vi "Get Resource Path.vi"(8 "Error In":errorcluster, 11 "Resource Filename":string="mine.PNG") -> (0 "Error Out":errorcluster, 3 "Resource Path":path)   [LabVIEW 2011]
doc: "Takes a filename, including file extension, of a file in the Resources directory of the built project and returns a filepath to that resource."
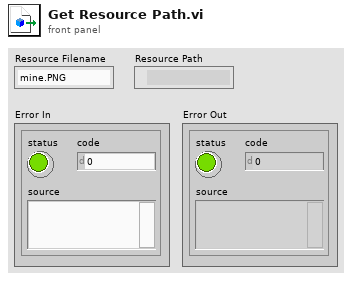
[diagram p1: front panel]
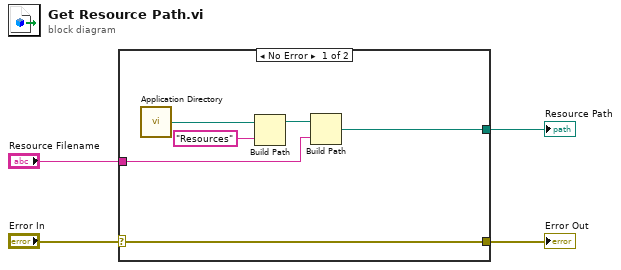
[diagram p0: block diagram]
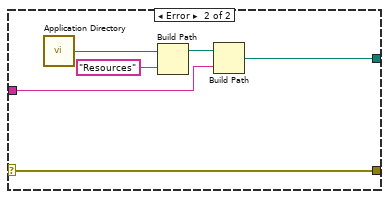
[diagram p2: hidden frame]
diagram:
  n1 = case shown="No Error" "Error In" {
    selector: "Error In" -> [w6 w11]
    tunnel: "Resource Filename" -> [w7 w12]
    tunnel: [w6 w11] -> w2
    tunnel: [w5 w13] -> w1
    frame No Error {
      n2 = call <vilib>:"Application Directory.vi"() -> ("Application Directory"=w9:path)
      n3 = Build Path(base path=w9, name or relative path="Resources") -> (appended path=w8:path)
      n4 = Build Path(base path=w8, name or relative path=w7) -> (appended path=w5:path)
    }
    frame Error {
      n5 = call <vilib>:"Application Directory.vi"() -> ("Application Directory"=w15:path)
      n6 = Build Path(base path=w15, name or relative path="Resources") -> (appended path=w14:path)
      n7 = Build Path(base path=w14, name or relative path=w12) -> (appended path=w13:path)
    }
  }
  "Error Out" <- w2
  "Resource Path" <- w1
